vi "From Variant.vi"(8 "error in (no error)":errorcluster, 10 "Variant":variant, 11 "Abs_String in":refnum<class "Abs_String.lvclass">) -> (0 "error out":errorcluster, 3 "Abs_String out":refnum<class "Abs_String.lvclass">)   [LabVIEW 2021, in "Abs_String.lvclass"]
uses:
  Abs_String.lvclass
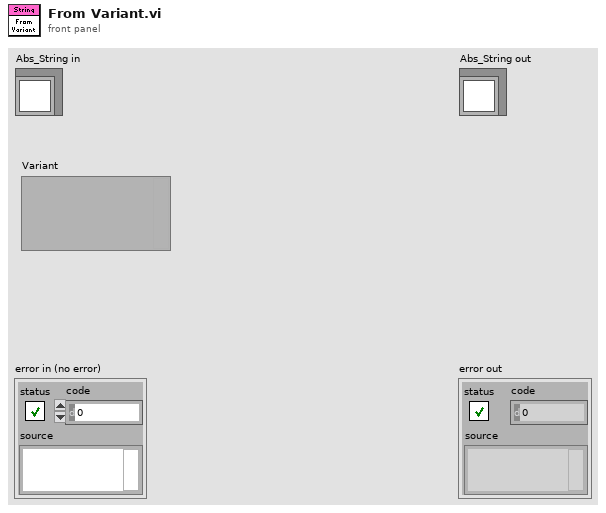
[diagram p1: front panel]
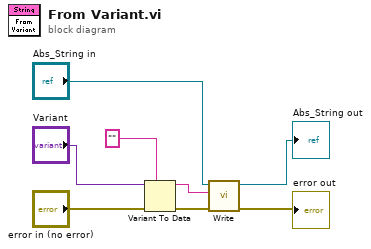
[diagram p0: block diagram]
diagram:
  n1 = Variant To Data(error in="error in (no error)", type="", Variant="Variant") -> (data=w5:string, error out=w6:errorcluster)
  n2 = call-dynamic "Write.vi"("error in (no error)"=w6, "String"=w5, "Abs_String in"="Abs_String in") -> ("error out"=→"error out":errorcluster, "Abs_String out"=→"Abs_String out":refnum<class "Abs_String.lvclass">)  [unwired: 7 in]
